vi "Write Value to Buffer.vi"(8 "error in (no error)":errorcluster, 10 "Value":variant, 11 "Timed Average Buffer":T1) -> (0 "error out":errorcluster, 1 "New Average Ready?":bool, 2 "Average":dbl, 3 "Timed Average Buffer":T1)   [LabVIEW 2015, in "TimedAverageBuffer.lvlib" / "TimedAverageBuffer.lvclass"]
uses:
  TimedAverageBuffer.lvclass
  TimedAverageBuffer Reference.ctl
  TimedAverageBuffer.lvclass/TimedAverageBuffer.ctl
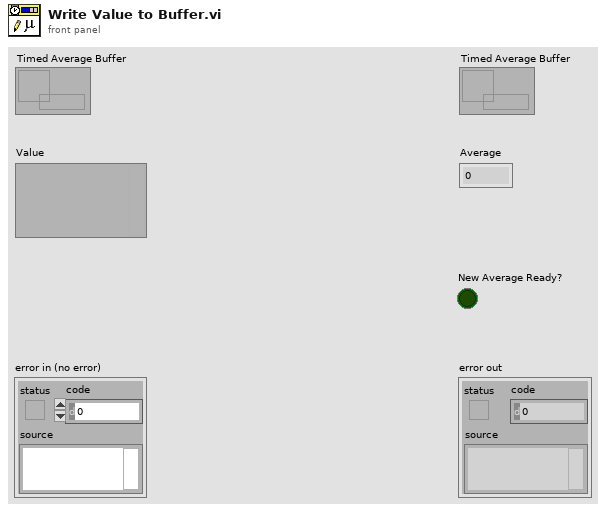
[diagram p1: front panel]
types:
  T1 = typedef "TimedAverageBuffer.lvlib/TimedAverageBuffer.lvclass/TimedAverageBuffer Reference.ctl" = refnum<data-value>
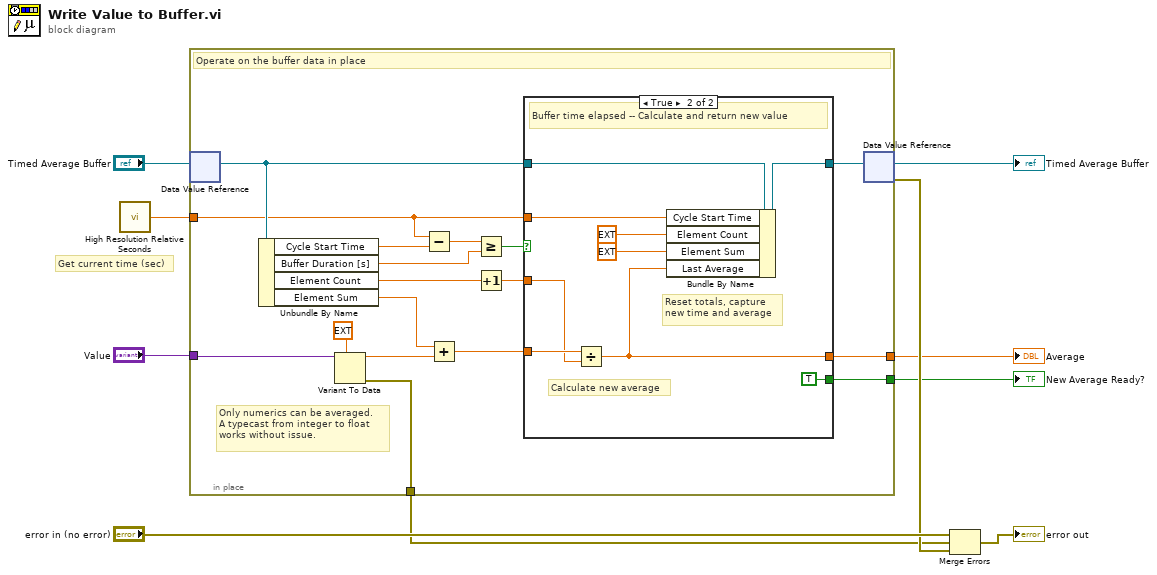
[diagram p0: block diagram]
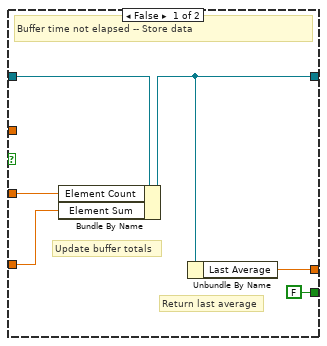
[diagram p2: hidden frame]
diagram:
  # "Get current time (sec)"
  n1 = call <vilib>:"High Resolution Relative Seconds.vi"() -> ("relative seconds"=w3:dbl)
  n2 = in-place {
    in-place-border: [w11] -> w5
    in-place-border: "Value" -> [w25]
    in-place-border: w3 -> [w16]
    in-place-border: [w18] -> w2
    in-place-border: [w17] -> w1
    # "Only numerics can be averaged.\nA typecast from integer to float\nworks without issue."
    # "Operate on the buffer data in place"
    n3 = in-place-dvr #1("Timed Average Buffer") -> (w27:refnum<class "TimedAverageBuffer.lvclass">)  [unwired: 1 out]
    n4 = Unbundle By Name(w27) -> ("Cycle Start Time"=w15:dbl, "Buffer Duration [s]"=w13:dbl, "Element Count"=w22:ext, "Element Sum"=w26:ext)
    n5 = Variant To Data(type=ext 0.0, Variant=w25) -> (data=w24:ext, error out=w11:errorcluster)  [unwired: 1 in]
    n6 = Subtract(x=w16, y=w15) -> (x-y=w14:dbl)
    n7 = Add(x=w26, y=w24) -> (x+y=w20:ext)
    n8 = Greater Or Equal?(x=w14, y=w13) -> (x >= y?=w12:bool)
    n9 = Increment(x=w22) -> (x+1=w19:ext)
    n10 = case shown="True" w12 {
      tunnel: w27 -> [w33 w42]
      tunnel: [w28 w41] -> w21
      tunnel: w20 -> [w31 w40]
      tunnel: w19 -> [w32 w39]
      tunnel: [w29 w34] -> w18
      tunnel: [FALSE TRUE] -> w17
      tunnel: w16 -> [_ w37]
      frame False {
        # "Return last average"
        # "Update buffer totals"
        # "Buffer time not elapsed -- Store data"
        n11 = Bundle By Name(cluster=w33, "Element Count"=w32, "Element Sum"=w31) -> (w28:refnum<class "TimedAverageBuffer.lvclass">)
        n12 = Unbundle By Name(w28) -> ("Last Average"=w29:dbl)
      }
      frame True {
        # "Reset totals, capture\nnew time and average"
        # "Calculate new average"
        # "Buffer time elapsed -- Calculate and return new value"
        n13 = Divide(x=w40, y=w39) -> (x/y=w34:dbl)
        n14 = Bundle By Name(cluster=w42, "Cycle Start Time"=w37, "Element Count"=ext 0.0, "Element Sum"=ext 0.0, "Last Average"=w34) -> (w41:refnum<class "TimedAverageBuffer.lvclass">)
      }
    }
    n15 = in-place-dvr #1(w21) -> (→"Timed Average Buffer":T1, w6:errorcluster)
  }
  "New Average Ready?" <- w1
  "Average" <- w2
  n16 = Merge Errors("error in (no error)", w5, w6) -> (→"error out":errorcluster)
